vi "X Listbox Update Symbols for Select.vi"(10 "Selected Row":i32, 11 "Number of Rows":u32) -> (3 "Item Symbols":i32[](array[numeric]))   [LabVIEW 2009]
doc: "This subVI is used in the creation of the facade for the X Listbox XControl.\n\nAAL 9/09"
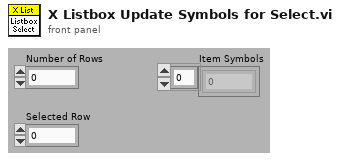
[diagram p1: front panel]
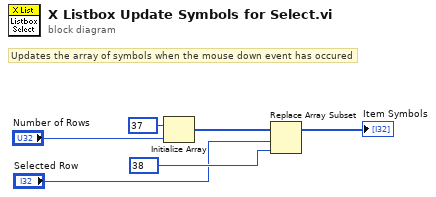
[diagram p0: block diagram]
diagram:
  # "Updates the array of symbols when the mouse down event has occured"
  n1 = Initialize Array(37, "Number of Rows") -> (w6:i32[])
  n2 = Replace Array Subset(array=w6, new element=38, index="Selected Row") -> (→"Item Symbols":i32[])
